vi "ToString.vi"(11 "Rectangle In":refnum<class "Rectangle.lvclass">) -> (2 "String":string, 3 "Rectangle Out":refnum<class "Rectangle.lvclass">)   [LabVIEW 2018, in "Rectangle.lvclass"]
uses:
  Rectangle.lvclass
  Rectangle.lvclass/Rectangle.ctl
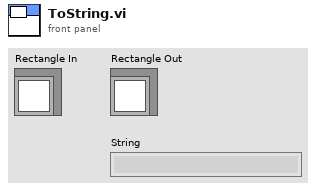
[diagram p1: front panel]
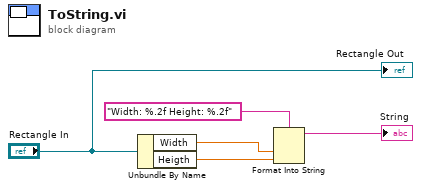
[diagram p0: block diagram]
diagram:
  n1 = Unbundle By Name("Rectangle In") -> ("Width"=w2:dbl, "Heigth"=w1:dbl)
  n2 = Format Into String(format string="Width: %.2f Height: %.2f", w2, w1) -> (resulting string=→"String":string)  [unwired: 2 in, 1 out]
  "Rectangle Out" <- "Rectangle In"
